vi "EXDIR-YAML_Dictionary_To_Predefined_Cluster.vi"(7 "Cluster Type":variant, 8 "error in (no error)":errorcluster, 9 "dictionary":T2) -> (0 "error out":errorcluster, 3 "VCluster out":variant)   [LabVIEW 2016]
uses:
  <userlib>/_OpenG.lib/dictionary/dictionary.llb/Dictionary Object RefNum__ogtk.ctl
  <userlib>/_OpenG.lib/dictionary/dictionary.llb/Dictionary Object RefNum - Enum__ogtk.ctl
  <vilib>/Utility/Data Type/Type Definitions/Data Type.ctl
  <userlib>/_OpenG.lib/string/string.llb/Trim Whitespace (String)__ogtk.vi
  <vilib>/Utility/Data Type/NI_Data Type.lvlib
panel:
  out "Type":T1
  out "Numeric":i32
  out "Array 2":variant[](array[variant])
  out "Array":T1[](array[typedef])
  out "hmm":string
  out "no badger box":variant
  out "empty box":variant
  out "items recieved":cluster{"key":variant, "value":variant}[](array[cluster])
  out "key in type cluster":string
  out "key":string
  out "Element Names":string[](array[string])
  out "Number of Elements":u16
  # "YAML parsing is close to working a little bit"
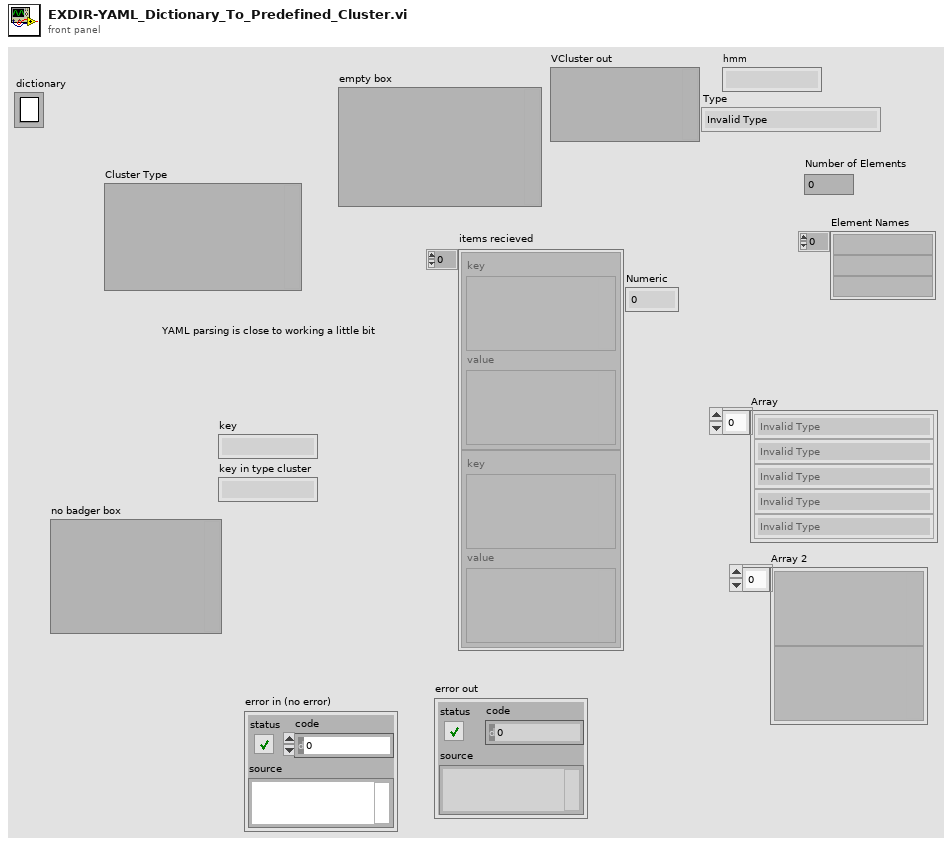
[diagram p1: front panel]
types:
  T1 = typedef "NI_Data Type.lvlib/Data Type.ctl" = enum8{"Invalid Type", "Void", "I8", "I16", "I32", "I64", "U8", "U16", "U32", "U64", "Single Float", "Double Float", "Extended Float", "Single Complex", "Double Complex", "Extended Complex", "Enum U8", "Enum U16", "Enum U32", "Enum U64", "Single Float With Unit", "Double Float With Unit", "Extended Float With Unit", "Single Complex with Unit", "Double Complex with Unit", "Extended Complex with Unit", "Boolean", "String", "Path", "Picture", "Tag", "Array", "Cluster", "Variant", "LV Variant", "Waveform", "Timestamp", "Digital Waveform", "Digital Data", "ExpressData", "Refnum", "External Data", "VI", "Poly VI", "LabVIEW Class Instance", "Fixed Point"}
  T2 = typedef "Dictionary Object RefNum__ogtk.ctl" = refnum<k1>
  T3 = enum32{"No Selection", "all ground", "all differential"}
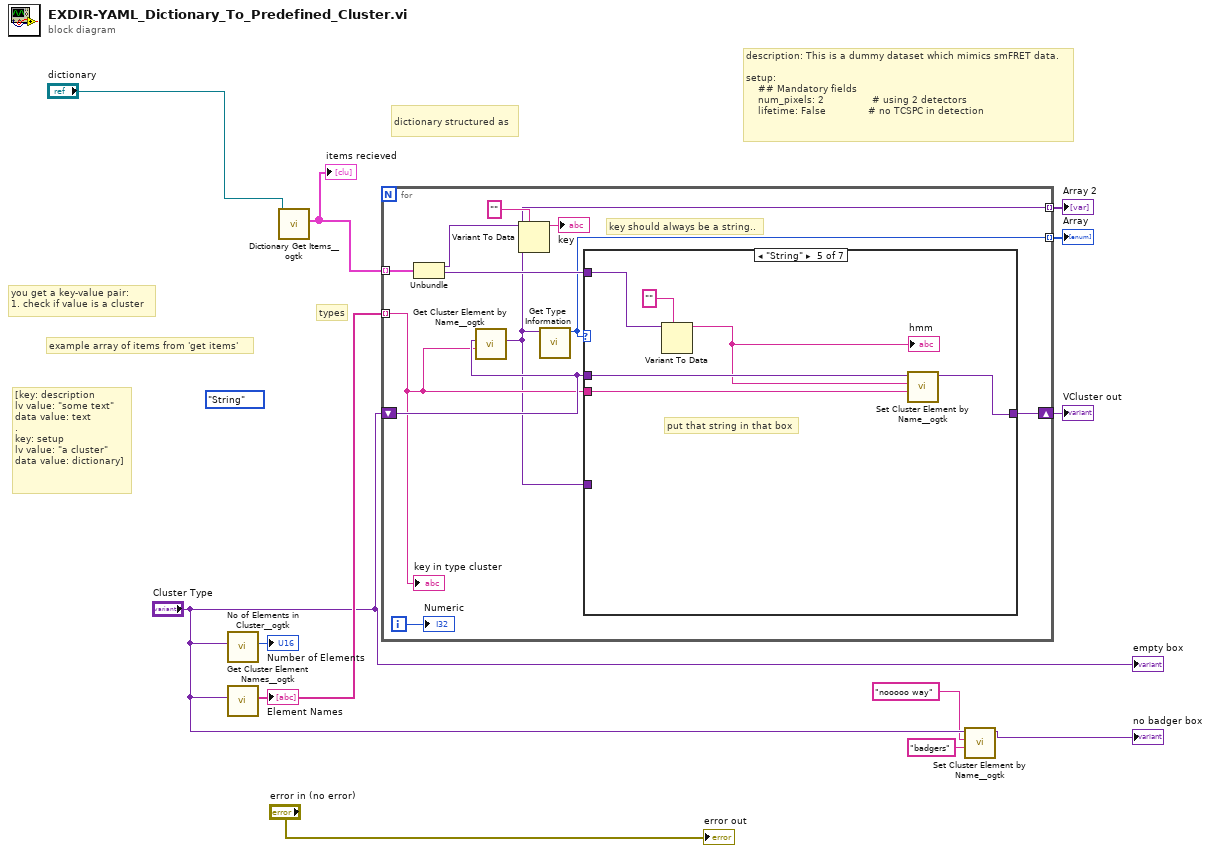
[diagram p0: block diagram]
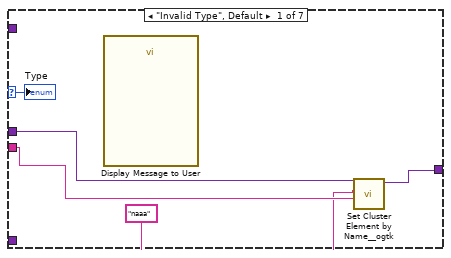
[diagram p2: hidden frame]
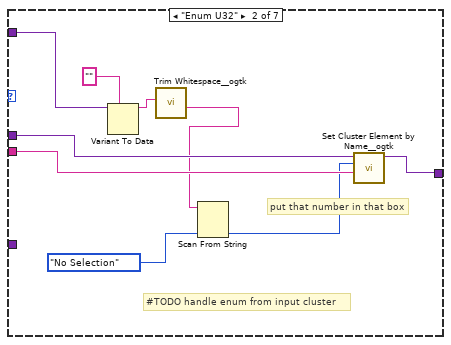
[diagram p3: hidden frame]
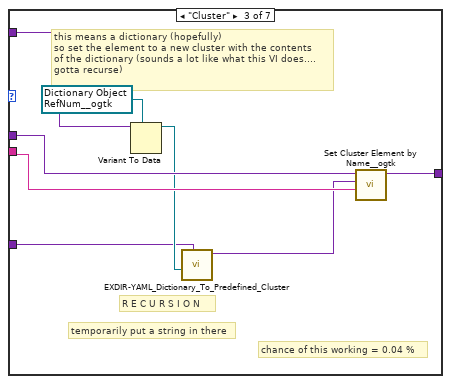
[diagram p4: hidden frame]
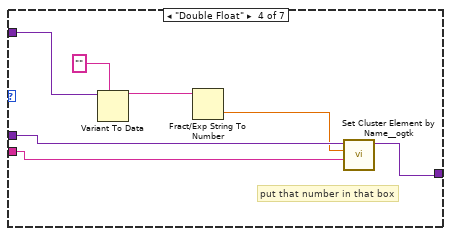
[diagram p5: hidden frame]
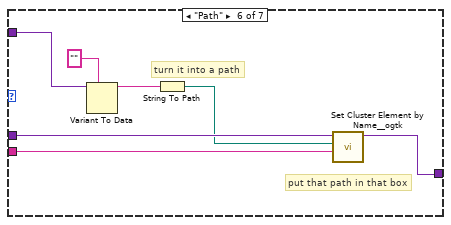
[diagram p6: hidden frame]
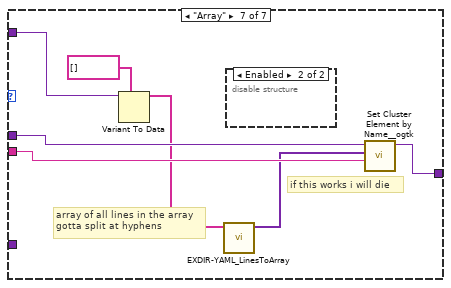
[diagram p7: hidden frame]
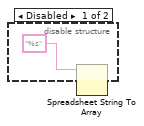
[diagram p8: hidden frame]
diagram:
  (unwired) Data_Type."String" ("Type")
  # "types"
  # "example array of items from 'get items'"
  # "[key: description\nlv value: \"some text\"\ndata value: text\n.\nkey: setup\nlv value: \"a cluster\"\ndata value: dictionary]"
  # "description: This is a dummy dataset which mimics smFRET data.\n\nsetup:\n    ## Mandatory fields\n    num_pixels: 2                # using 2 detectors\n    lifetime: False              # no TCSPC in detection"
  # "you get a key-value pair:\n1. check if value is a cluster"
  # "dictionary structured as"
  n1 = call <userlib>:"No of Elements in Cluster__ogtk.vi"("Cluster"="Cluster Type") -> ("Number of Elements"=→"Number of Elements":u16)  [unwired: 9 in, 1 out]
  n2 = call <userlib>:"Get Cluster Element Names__ogtk.vi"("Cluster"="Cluster Type") -> ("Element Names"=w10:string[])  [unwired: 9 in, 1 out]
  "Element Names" <- w10
  n3 = call <userlib>:"Dictionary Get Items__ogtk.vi"("dictionary"="dictionary") -> ("items"=w9:cluster{"key":variant, "value":variant}[])  [unwired: 8 in, 2 out]
  "items recieved" <- w9
  n4 = for {
    tunnel: w9 -> [w23] mode=indexing
    tunnel: w10 -> [w16] mode=indexing
    tunnel: [w15] -> w3 mode=indexing
    tunnel: [w14] -> w2 mode=indexing
    shift-right: [w18] -> w4
    shift-left: "Cluster Type" -> [w17]
    i -> [w13]
    # "key should always be a string.."
    n5 = Unbundle(w23) -> ("key"=w21:variant, "value"=w19:variant)
    n6 = call <userlib>:"Get Cluster Element by Name__ogtk.vi"("Element Name"=w16, "Cluster"=w17) -> ("VElement"=w14:variant)  [unwired: 7 in, 2 out]
    n7 = Variant To Data(type="", Variant=w21) -> (data=→"key":string)  [unwired: 1 in, 1 out]
    n8 = call <vilib>:"Get Type Information.vi"("Variant"=w14) -> ("Type"=w15:T1)  [unwired: 6 in, 4 out]
    n9 = case shown="\"String\"" w15 {
      selector: w15 -> [w24 _ _ _ _ _ _]
      tunnel: w16 -> [w28 w35 w45 w51 w58 w65 w70]
      tunnel: w17 -> [w27 w36 w44 w52 w57 w64 w71]
      tunnel: w19 -> [_ w34 w42 w50 w56 w63 w69]
      tunnel: [w26 w31 w43 w49 w54 w62 w72] -> w18
      tunnel: w14 -> [_ _ w39 _ _ _ _]
      frame "Invalid Type", Default {
        n10 = call "Display Message to User"() -> ()  [unwired: 10 in, 2 out]
        n11 = call <userlib>:"Set Cluster Element by Name__ogtk.vi"("Element Name (\"\": New Element Data Name)"=w28, "New Element Value"="naaa", "Cluster"=w27) -> ("VCluster out"=w26:variant)  [unwired: 6 in, 2 out]
        "Type" <- w24
      }
      frame "Enum U32" {
        # "#TODO handle enum from input cluster"
        # "put that number in that box"
        n12 = Variant To Data(type="", Variant=w34) -> (data=w33:string)  [unwired: 1 in, 1 out]
        n13 = call-poly <userlib>:"Trim Whitespace__ogtk.vi"("String in"=w33) -> ("String out"=w30:string)  [unwired: 6 in]
        n14 = Scan From String(input string=w30, default 1=T3."No Selection" ("Radio Buttons")) -> (output 1=w32:T3)  [unwired: 3 in, 3 out]
        n15 = call <userlib>:"Set Cluster Element by Name__ogtk.vi"("Element Name (\"\": New Element Data Name)"=w35, "New Element Value"=w32, "Cluster"=w36) -> ("VCluster out"=w31:variant)  [unwired: 6 in, 2 out]
      }
      frame "Cluster" {
        w41 = T2 refnum items=["Dictionary"] ("dictionary")
        # "chance of this working = 0.04 %"
        # "R E C U R S I O N"
        # "temporarily put a string in there"
        # "this means a dictionary (hopefully)\nso set the element to a new cluster with the contents\nof the dictionary (sounds a lot like what this VI does....\ngotta recurse)"
        n16 = Variant To Data(type=w41, Variant=w42) -> (data=w40:T2)  [unwired: 1 in, 1 out]
        n17 = call "EXDIR-YAML_Dictionary_To_Predefined_Cluster.vi"("Cluster Type"=w39, "dictionary"=w40) -> ("VCluster out"=w38:variant)  [unwired: 8 in, 1 out]
        n18 = call <userlib>:"Set Cluster Element by Name__ogtk.vi"("Element Name (\"\": New Element Data Name)"=w45, "New Element Value"=w38, "Cluster"=w44) -> ("VCluster out"=w43:variant)  [unwired: 6 in, 2 out]
      }
      frame "Double Float" {
        # "put that number in that box"
        n19 = Variant To Data(type="", Variant=w50) -> (data=w47:string)  [unwired: 1 in, 1 out]
        n20 = Fract/Exp String To Number(string=w47) -> (number=w46:dbl)  [unwired: 3 in, 1 out]
        n21 = call <userlib>:"Set Cluster Element by Name__ogtk.vi"("Element Name (\"\": New Element Data Name)"=w51, "New Element Value"=w46, "Cluster"=w52) -> ("VCluster out"=w49:variant)  [unwired: 6 in, 2 out]
      }
      frame "String" {
        # "put that string in that box"
        n22 = Variant To Data(type="", Variant=w56) -> (data=w55:string)  [unwired: 1 in, 1 out]
        "hmm" <- w55
        n23 = call <userlib>:"Set Cluster Element by Name__ogtk.vi"("Element Name (\"\": New Element Data Name)"=w58, "New Element Value"=w55, "Cluster"=w57) -> ("VCluster out"=w54:variant)  [unwired: 6 in, 2 out]
      }
      frame "Path" {
        # "put that path in that box"
        # "turn it into a path"
        n24 = Variant To Data(type="", Variant=w63) -> (data=w60:string)  [unwired: 1 in, 1 out]
        n25 = String To Path(string=w60) -> (path=w59:path)
        n26 = call <userlib>:"Set Cluster Element by Name__ogtk.vi"("Element Name (\"\": New Element Data Name)"=w65, "New Element Value"=w59, "Cluster"=w64) -> ("VCluster out"=w62:variant)  [unwired: 6 in, 2 out]
      }
      frame "Array" {
        # "array of all lines in the array\ngotta split at hyphens"
        # "if this works i will die"
        n27 = Variant To Data(type=string[] [], Variant=w69) -> (data=w67:string[])  [unwired: 1 in, 1 out]
        n28 = call "EXDIR-YAML_LinesToArray.vi"("array of lines in"=w67) -> ("Array"=w66:variant[])  [unwired: 9 in, 1 out]
        n29 = disable-structure shown="Enabled" {
          frame Disabled {
            n30 = Spreadsheet String To Array(format string="%s") -> ()  [unwired: 3 in, 1 out]
          }
          frame Enabled {
          }
        }
        n31 = call <userlib>:"Set Cluster Element by Name__ogtk.vi"("Element Name (\"\": New Element Data Name)"=w70, "New Element Value"=w66, "Cluster"=w71) -> ("VCluster out"=w72:variant)  [unwired: 6 in, 2 out]
      }
    }
    "key in type cluster" <- w16
    "Numeric" <- w13
  }
  "VCluster out" <- w4
  "Array" <- w3
  "Array 2" <- w2
  n32 = call <userlib>:"Set Cluster Element by Name__ogtk.vi"("Element Name (\"\": New Element Data Name)"="badgers" ("Element Name (\"\": New Element Data Name)"), "New Element Value"="nooooo way", "Cluster"="Cluster Type") -> ("VCluster out"=→"no badger box":variant)  [unwired: 6 in, 2 out]
  "empty box" <- "Cluster Type"
  "error out" <- "error in (no error)"
